vi "Sonar_cm_mod.vi"(2 "NXT":T2={"Hardware"="NXT", "Flattened String"=""}, 3 "Port (Port 4)":T1=3 items=["Port 1", "Port 2", "Port 3", "Port 4"]) -> (1 "Distance (cm)":i16, 4 "NXT":T2={"Hardware"="NXT", "Flattened String"=""})   [LabVIEW 2011]
doc: "Reads the ultrasonic sensor connected to the specified input port and outputs the distance in centimeters.\n\n<B>Inputs\nNXT </B> connects to NXT terminal of previous VI to establish the flow of the program.\n<B>Port (Port 4) </B> is the port connected to the ultrasonic sensor. Port 4 is the default, but Port 1, Port 2, or Port 3 can also be selected.\n\n<B>Outputs\nNXT </B> wires to NXT terminal of next VI to establish the flow of the program.\n<B>Distance (cm)</B> returns the value of the distance sensor (cm)."
uses:
  <vilib>/NXT/Subs/LVHSConnector.ctl
  <vilib>/NXT/Block Support/NXT_InputPort.ctl
  <vilib>/NXT/Block Support/HWPage.SensorType.ctl
  <vilib>/NXT/Block Support/HWPage.SensorMode.ctl
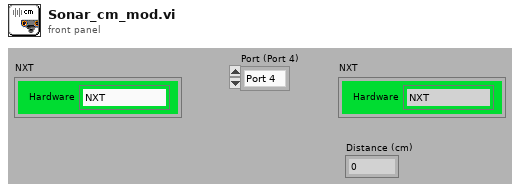
[diagram p1: front panel]
types:
  T1 = typedef "NXT_InputPort.ctl" = u8
  T2 = typedef "LVHSConnector.ctl" = cluster{"Hardware":string, "Flattened String":string}
  T3 = typedef "HWPage.SensorType.ctl" = u8
  T4 = typedef "HWPage.SensorMode.ctl" = u8
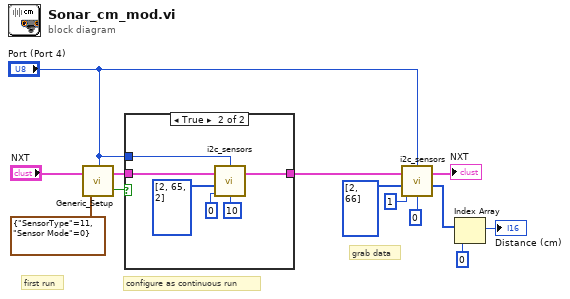
[diagram p0: block diagram]
diagram:
  # "configure as continuous run"
  # "first run"
  # "grab data"
  n1 = call <vilib>:"Generic_Setup.vi"("Sensor Setup"=cluster{"SensorType":T3, "Sensor Mode":T4} {"SensorType"=11, "Sensor Mode"=0}, "NXT"="NXT", "Port"="Port (Port 4)") -> ("Changed?"=w2:bool, "NXT"=w3:T2)
  n2 = case shown="True" w2 {
    tunnel: w3 -> [w14 w20]
    tunnel: [w14 w15] -> w4
    tunnel: "Port (Port 4)" -> [_ w19]
    frame False {
    }
    frame True {
      n3 = call <vilib>:"i2c_sensors.vi"("Return Length"=u8 0, "Bytes to Write"=u8[] [2, 65, 2] ("Buffer"), "Wait (msec)"=u32 10, "NXT"=w20, "Port"=w19) -> ("NXT"=w15:T2)  [unwired: 2 out]
    }
  }
  n4 = call <vilib>:"i2c_sensors.vi"("Return Length"=u8 1, "Bytes to Write"=u8[] [2, 66] ("Parameters"), "Wait (msec)"=u32 0, "NXT"=w4, "Port"="Port (Port 4)") -> ("Bytes read"=w10:u8[], "NXT"=→"NXT":T2)  [unwired: 1 out]
  n5 = Index Array(array=w10, index=0) -> (element=→"Distance (cm)":u8)
